vi "filter pipe.vi"(0 "omega  in":dbl[](array[numeric]), 2 "z in":cdb[](array[numeric]), 3 "upper":dbl=0.07, 5 "lower":dbl=0.01, 7 "Plot: complex plane - filter":refnum<vi>, 8 "filter using":T1(ring), 9 "interpolated omega (kHz)":dbl, 10 "filter window (kHz)":dbl=40.0 caption="(kHz)", 11 "interpolated gamma (kHz)":dbl) -> (14 "omega out":dbl[](array[numeric]), 16 "z out":cdb[](array[numeric]), 17 "center":cdb, 18 "norm":dbl, 19 "filter w (kHz)":dbl)   [LabVIEW 2010]
uses:
  <vilib>/Analysis/6fits.llb/Curve Fitting Criteria.ctl
  <vilib>/Analysis/3filter.llb/Filter Passband Type.ctl
  tale of three indices -- selector -- control.ctl
  tale of three indices -- int -- control.ctl
  linear interpolation - complex.vi
  Q -- check range -- i -- integer.vi
  command stack.vi
  generate linear region.vi
  <vilib>/Analysis/NI_AALPro.lvlib
  <vilib>/Analysis/NI_AALBase.lvlib
  <vilib>/Analysis/3filter.llb/FIR Windowed Filter (DBL).vi
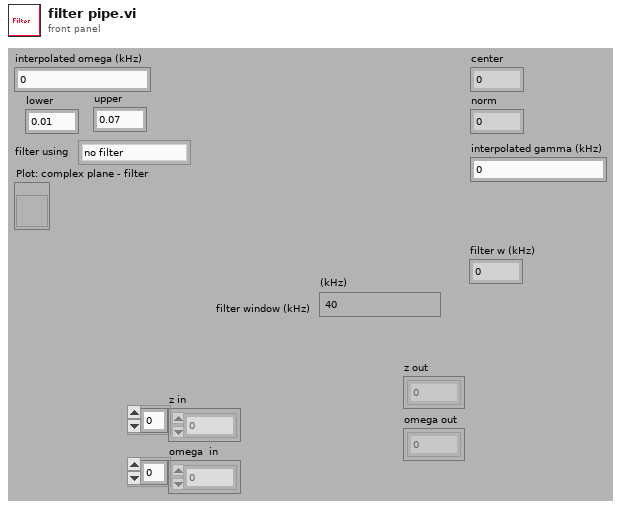
[diagram p1: front panel]
types:
  T1 = enum16{"no filter", "median", "liner fit on median", "interpolation", "smart interpolation"}
  T2 = typedef "NI_AALBase.lvlib/Filter Passband Type.ctl" = enum32{"Lowpass", "Highpass", "Bandpass", "Bandstop"}
  T3 = typedef "tale of three indices -- selector -- control.ctl" = enum16{"window right", "window left", "balance", "shrink", "broaden", "do nothing", "reset", "center right", "center left", "all left", "all right", "check"}
  T4 = typedef "NI_AALPro.lvlib/Curve Fitting Criteria.ctl" = u16
  T5 = typedef "tale of three indices -- int -- control.ctl" = cluster{"left":i32, "center":i32, "right":i32, "right most":i32, "left most":i32, "window":i32}
  T6 = typedef "comparison control.ctl" = enum16{"not a number", "above", "in range", "below"}
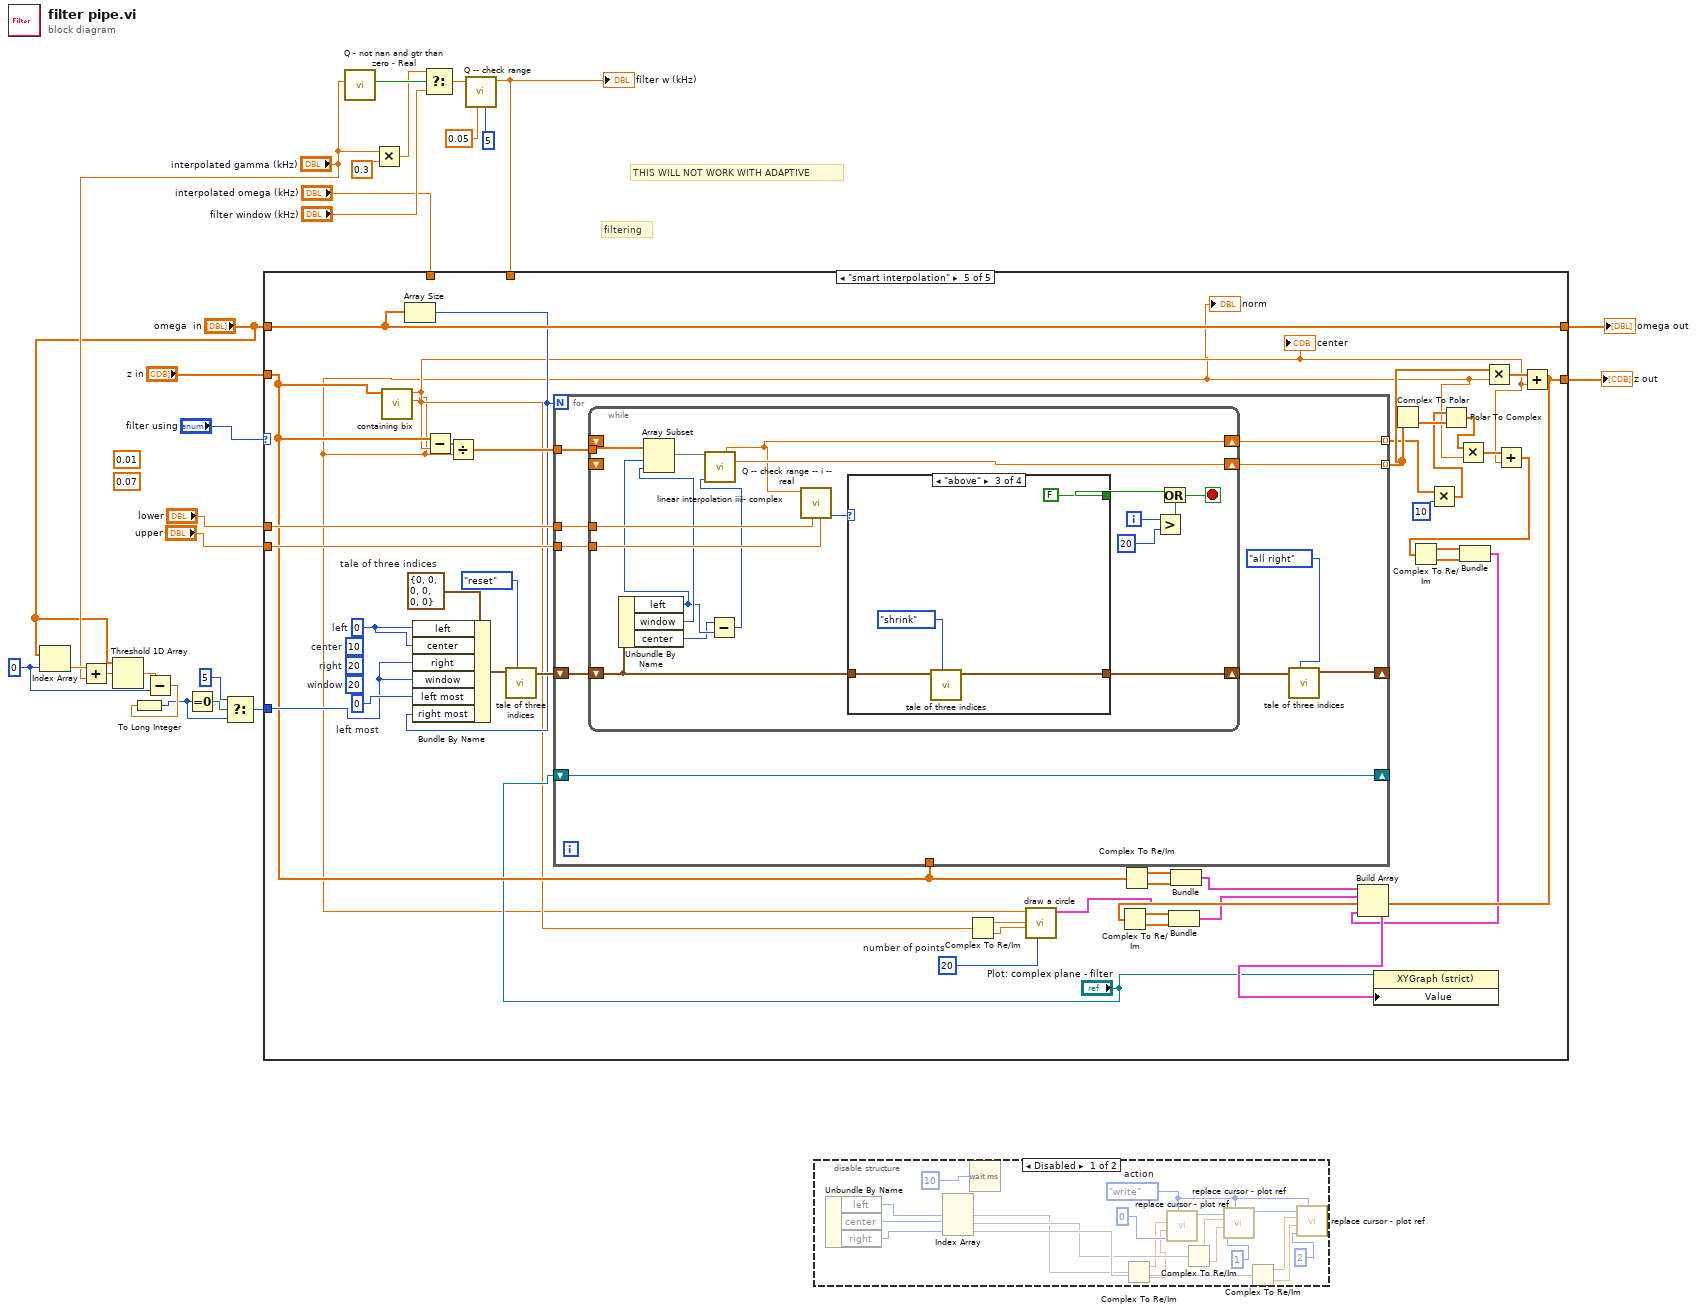
[diagram p0: block diagram]
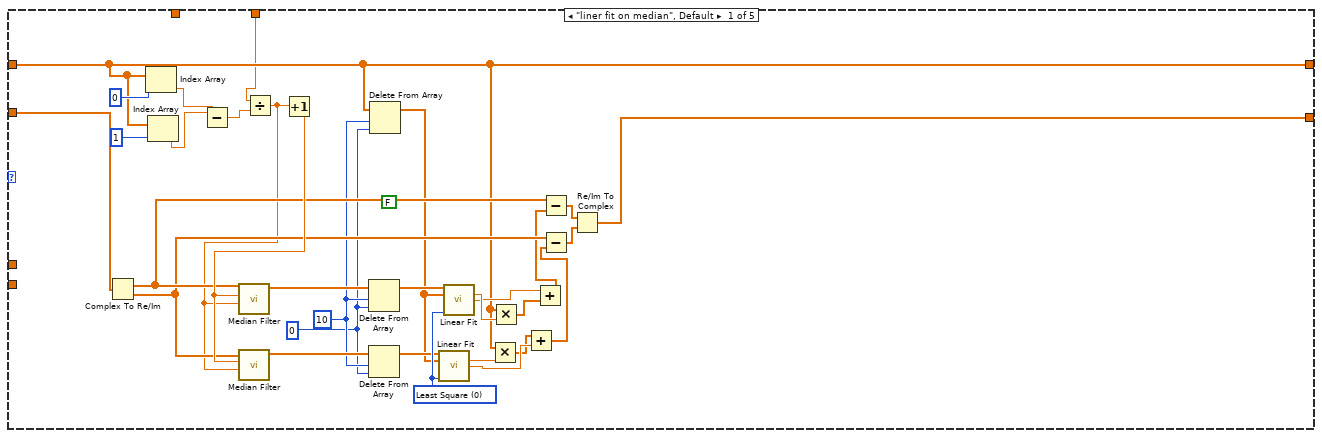
[diagram p3: hidden frame]
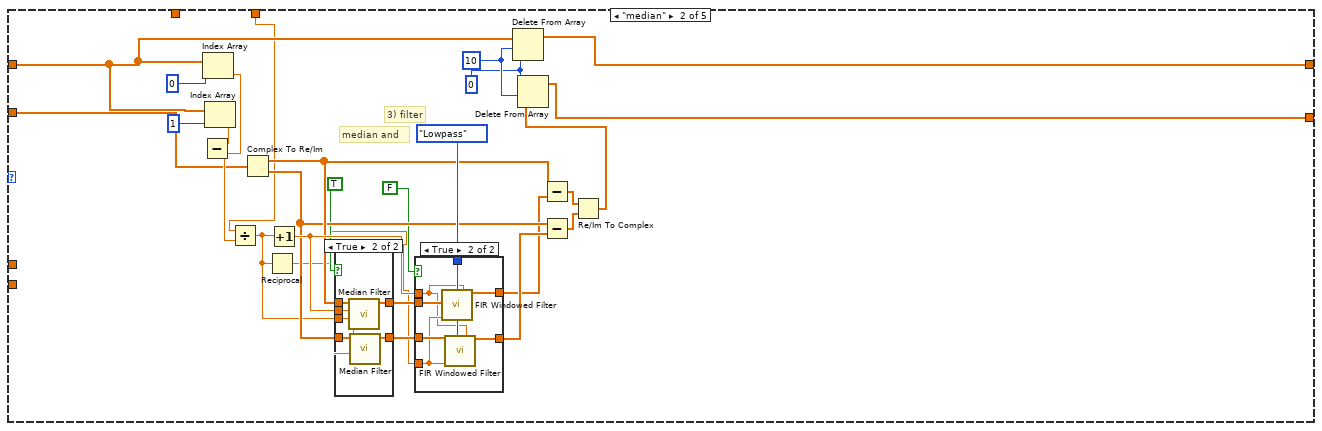
[diagram p4: hidden frame]
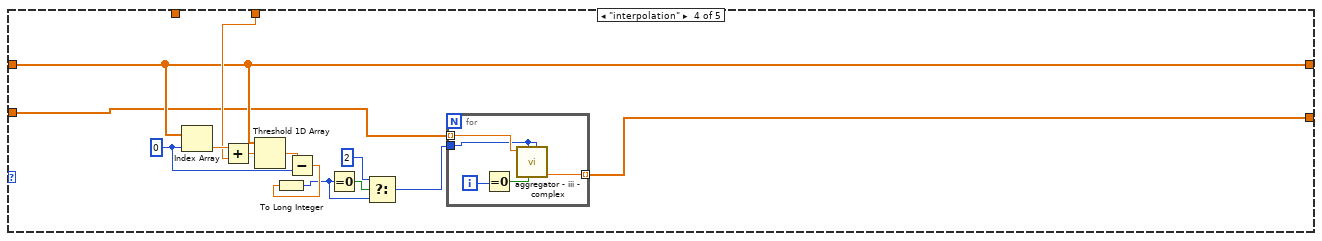
[diagram p8: hidden frame]
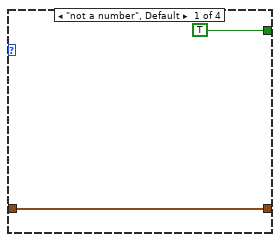
[diagram p9: hidden frame]
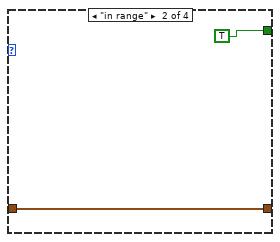
[diagram p10: hidden frame]
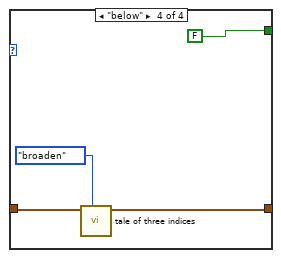
[diagram p11: hidden frame]
diagram:
  (unwired) 0.07
  (unwired) 0.01
  w10 = 0 ("index")
  # "THIS WILL NOT WORK WITH ADAPTIVE"
  # "filtering"
  n1 = Index Array(array="omega  in", index=w10) -> (element=w13:dbl)
  n2 = Add(x=w13, y="interpolated gamma (kHz)") -> (x+y=w12:dbl)
  n3 = Threshold 1D Array(2:w12, 3:"omega  in") -> (0:w11:dbl)  [unwired: 1 in]
  n4 = Subtract(x=w11, y=w10) -> (x-y=w9:dbl)
  n5 = To Long Integer(number=w9) -> (32bit integer=w6:i32)
  n6 = Equal To 0?(x=w6) -> (x = 0?=w8:bool)
  n7 = Select(t=5, s=w8, f=w6) -> (s? t:f=w4:i32)
  n8 = call "Q - not nan and gtr than zero - Real.vi"("Numeric"="interpolated gamma (kHz)") -> ("Boolean"=w22:bool)  [unwired: 9 in, 1 out]
  n9 = Multiply(x="interpolated gamma (kHz)", y=0.3) -> (x*y=w21:dbl)
  n10 = Select(t=w21, s=w22, f="filter window (kHz)") -> (s? t:f=w18:dbl)
  n11 = call "Q -- check range.vi"("upper"=5, "lower"=0.05, "number"=w18) -> ("number in range"=w17:dbl)  [unwired: 4 in, 4 out]
  "filter w (kHz)" <- w17
  n12 = case shown="\"smart interpolation\"" "filter using" {
    tunnel: "omega  in" -> [w29 w64 w103 w114 w162]
    tunnel: [w45 w65 w102 w108 w145] -> w24
    tunnel: "z in" -> [w47 w70 w102 w109 w137]
    tunnel: [w29 w61 w103 w114 w162] -> w25
    tunnel: w17 -> [w27 w58 _ w115 _]
    tunnel: "interpolated omega (kHz)" -> [_ _ _ _ _]
    tunnel: w4 -> [_ _ _ _ w153]
    tunnel: "lower" -> [_ _ _ _ w158]
    tunnel: "upper" -> [_ _ _ _ w157]
    frame "liner fit on median", Default {
      w39 = 0 ("index")
      w40 = 10 ("length")
      w46 = T4 0 items=["Least Square", "Least Absolute Residual", "Bisquare"] ("method")
      (unwired) FALSE
      n13 = Complex To Re/Im(x + iy=w47) -> (x=w50:dbl[], y=w49:dbl[])
      n14 = Index Array(array=w29, index=0) -> (element=w28:dbl)
      n15 = Index Array(array=w29, index=1) -> (element=w53:dbl)
      n16 = Subtract(x=w53, y=w28) -> (x-y=w52:dbl)
      n17 = Divide(x=w27, y=w52) -> (x/y=w48:dbl)
      n18 = Increment(x=w48) -> (x+1=w51:dbl)
      n19 = call <vilib>:"Median Filter.vi"("right rank"=w48, "left rank"=w51, "X"=w50) -> ("Filtered X"=w44:dbl[])  [unwired: 7 in, 1 out]
      n20 = call <vilib>:"Median Filter.vi"("right rank"=w48, "left rank"=w51, "X"=w49) -> ("Filtered X"=w41:dbl[])  [unwired: 7 in, 1 out]
      n21 = Delete From Array(array=w44, length=w40, index=w39) -> (array with subset deleted=w43:dbl[])  [unwired: 1 out]
      n22 = Delete From Array(array=w41, length=w40, index=w39) -> (array with subset deleted=w42:dbl[])  [unwired: 1 out]
      n23 = Delete From Array(array=w29, length=w40, index=w39) -> (array with subset deleted=w38:dbl[])  [unwired: 1 out]
      n24 = call <vilib>:"Linear Fit.vi"("Y"=w42, "X"=w38, "method"=w46) -> ("slope"=w35:dbl, "intercept"=w34:dbl)  [unwired: 8 in, 3 out]
      n25 = call <vilib>:"Linear Fit.vi"("Y"=w43, "X"=w38, "method"=w46) -> ("slope"=w36:dbl, "intercept"=w33:dbl)  [unwired: 8 in, 3 out]
      n26 = Multiply(x=w29, y=w35) -> (x*y=w32:dbl[])
      n27 = Multiply(x=w29, y=w36) -> (x*y=w37:dbl[])
      n28 = Add(x=w32, y=w34) -> (x+y=w31:dbl[])
      n29 = Add(x=w33, y=w37) -> (x+y=w30:dbl[])
      n30 = Subtract(x=w50, y=w30) -> (x-y=w57:dbl[])
      n31 = Subtract(x=w49, y=w31) -> (x-y=w56:dbl[])
      n32 = Re/Im To Complex(1:w56, 2:w57) -> (0:w45:cdb[])
    }
    frame "median" {
      w62 = 0 ("index")
      w63 = 10 ("length")
      # "median and"
      # "3) filter"
      n33 = Index Array(array=w64, index=0) -> (element=w79:dbl)
      n34 = Index Array(array=w64, index=1) -> (element=w80:dbl)
      n35 = Subtract(x=w80, y=w79) -> (x-y=w78:dbl)
      n36 = Divide(x=w58, y=w78) -> (x/y=w69:dbl)
      n37 = Complex To Re/Im(x + iy=w70) -> (x=w72:dbl[], y=w71:dbl[])
      n38 = Reciprocal(x=w69) -> (1/x=w59:dbl)
      n39 = Increment(x=w69) -> (x+1=w73:dbl)
      n40 = case shown="True" TRUE {
        tunnel: [w86 w92] -> w77
        tunnel: [w85 w91] -> w76
        tunnel: w73 -> [_ w90]
        tunnel: w72 -> [w86 w89]
        tunnel: w71 -> [w85 w88]
        tunnel: w69 -> [_ w87]
        frame False {
        }
        frame True {
          n41 = call <vilib>:"Median Filter.vi"("right rank"=w87, "left rank"=w90, "X"=w89) -> ("Filtered X"=w92:dbl[])  [unwired: 7 in, 1 out]
          n42 = call <vilib>:"Median Filter.vi"("right rank"=w87, "left rank"=w90, "X"=w88) -> ("Filtered X"=w91:dbl[])  [unwired: 7 in, 1 out]
        }
      }
      n43 = case shown="True" FALSE {
        tunnel: w77 -> [w94 w101]
        tunnel: [w94 w100] -> w60
        tunnel: w76 -> [w93 w99]
        tunnel: [w93 w98] -> w75
        tunnel: Filter_Passband_Type."Lowpass" ("filter type") -> [_ w97]
        tunnel: w59 -> [_ w96]
        tunnel: w73 -> [_ w95]
        frame False {
        }
        frame True {
          n44 = call-poly <vilib>:"FIR Windowed Filter.vi"("X"=w101, "filter type"=w97, "window parameter"=w95, "high cutoff freq: fh"=w96) -> ("Filtered X"=w100:dbl[])  [unwired: 10 in, 1 out]
          n45 = call-poly <vilib>:"FIR Windowed Filter.vi"("X"=w99, "filter type"=w97, "window parameter"=w95, "high cutoff freq: fh"=w96) -> ("Filtered X"=w98:dbl[])  [unwired: 10 in, 1 out]
        }
      }
      n46 = Delete From Array(array=w64, length=w63, index=w62) -> (array with subset deleted=w61:dbl[])  [unwired: 1 out]
      n47 = Subtract(x=w72, y=w60) -> (x-y=w84:dbl[])
      n48 = Subtract(x=w71, y=w75) -> (x-y=w83:dbl[])
      n49 = Re/Im To Complex(1:w83, 2:w84) -> (0:w66:cdb[])
      n50 = Delete From Array(array=w66, length=w63, index=w62) -> (array with subset deleted=w65:cdb[])  [unwired: 1 out]
    }
    frame "no filter" {
    }
    frame "interpolation" {
      w111 = 0 ("index")
      n51 = Index Array(array=w114, index=w111) -> (element=w116:dbl)
      n52 = Add(x=w116, y=w115) -> (x+y=w113:dbl)
      n53 = Threshold 1D Array(2:w113, 3:w114) -> (0:w112:dbl)  [unwired: 1 in]
      n54 = Subtract(x=w112, y=w111) -> (x-y=w110:dbl)
      n55 = To Long Integer(number=w110) -> (32bit integer=w105:i32)
      n56 = Equal To 0?(x=w105) -> (x = 0?=w107:bool)
      n57 = Select(t=2, s=w107, f=w105) -> (s? t:f=w104:i32)
      n58 = for {
        tunnel: w104 -> [w120]
        tunnel: w109 -> [w121] mode=indexing
        tunnel: [w117] -> w108 mode=indexing
        i -> [w119]
        n59 = Equal To 0?(x=w119) -> (x = 0?=w118:bool)
        n60 = call "aggregator - iii - complex.vi"("requested averaging interval"=w120, "first time"=w118, "requested size"=w120, "number"=w121) -> ("interpolated average"=w117:cdb)  [unwired: 3 in, 4 out]
      }
    }
    frame "smart interpolation" {
      w140 = 20  # number of points
      w156 = T5 {"left"=0, "center"=0, "right"=0, "right most"=0, "left most"=0, "window"=0}  # tale of three indices
      w155 = 0  # left most
      (unwired) 20  # window
      (unwired) 20  # right
      w154 = 0  # left
      (unwired) 10  # center
      n61 = call "containing bix.vi"("z in"=w137) -> ("norm"=w122:dbl, "center"=w130:cdb)  [unwired: 9 in]
      "center" <- w130
      "norm" <- w122
      n62 = Array Size(array=w162) -> (size(s)=w150:i32)
      n63 = Bundle By Name(cluster=w156, "left"=w154, "center"=w154, "right"=w153, "window"=w153, "left most"=w155, "right most"=w150) -> (w152:T5)
      n64 = Subtract(x=w137, y=w130) -> (x-y=w161:cdb[])
      n65 = Divide(x=w161, y=w122) -> (x/y=w160:cdb[])
      n66 = call "tale of three indices.vi"("selector"=tale_of_three_indices_--_selector_--_control."reset", "tale of three indices -- int -- control"=w152) -> ("tale of three indices -- int -- control out"=w159:T5)  [unwired: 6 in, 3 out]
      n67 = for {
        N: w150 -> [_]
        shift-right: [w167] -> _
        shift-left: w159 -> [w166]
        tunnel: [w172] -> w134 mode=indexing
        tunnel: w160 -> [w165]
        tunnel: w158 -> [w171]
        tunnel: w157 -> [w170]
        tunnel: w137 -> [_]
        shift-right: [w164] -> _
        shift-left: "Plot: complex plane - filter" -> [w164]
        tunnel: [w163] -> w125 mode=indexing
        n68 = while {
          tunnel: w165 -> [w189]
          shift-right: [w186] -> w168
          shift-left: w166 -> [w178]
          tunnel: w171 -> [w180]
          tunnel: w170 -> [w179]
          shift-right: [w173] -> w163
          shift-left: _ -> [_]
          shift-right: [w188] -> w172
          shift-left: _ -> [_]
          i -> [w183]
          stop <- w185 stop-if-true
          n69 = Unbundle By Name(w178) -> ("left"=w176:i32, "window"=w177:i32, "center"=w175:i32)
          n70 = Array Subset(array=w189, index=w176, length=w177) -> (w190:cdb[])
          n71 = Subtract(x=w175, y=w176) -> (x-y=w174:i32)
          n72 = call "linear interpolation iiii- complex.vi"("Array"=w190, "center"=w174) -> ("directed sigma"=w173:dbl, "center"=w188:cdb)  [unwired: 5 in, 7 out]
          n73 = call "Q -- check range -- i -- real.vi"("upper"=w179, "lower"=w180, "number"=w173) -> ("selector"=w187:T6)  [unwired: 6 in, 2 out]
          n74 = case shown="\"above\"" w187 {
            tunnel: [TRUE TRUE FALSE FALSE] -> w184
            tunnel: [w191 w194 w196 w199] -> w186
            tunnel: w178 -> [w191 w194 w197 w200]
            frame "not a number", Default {
            }
            frame "in range" {
            }
            frame "above" {
              n75 = call "tale of three indices.vi"("selector"=tale_of_three_indices_--_selector_--_control."shrink", "tale of three indices -- int -- control"=w197) -> ("tale of three indices -- int -- control out"=w196:T5)  [unwired: 6 in, 3 out]
            }
            frame "below" {
              n76 = call "tale of three indices.vi"("selector"=tale_of_three_indices_--_selector_--_control."broaden", "tale of three indices -- int -- control"=w200) -> ("tale of three indices -- int -- control out"=w199:T5)  [unwired: 6 in, 3 out]
            }
          }
          n77 = Greater?(x=w183, y=20) -> (0:w181:bool)
          n78 = Or(x=w184, y=w181) -> (x .or. y?=w185:bool)
        }
        n79 = call "tale of three indices.vi"("selector"=tale_of_three_indices_--_selector_--_control."all right", "tale of three indices -- int -- control"=w168) -> ("tale of three indices -- int -- control out"=w167:T5)  [unwired: 6 in, 3 out]
      }
      n80 = Complex To Re/Im(x + iy=w130) -> (x=w142:dbl, y=w141:dbl)
      n81 = call "draw a circle.vi"("number of points"=w140, "center Y"=w141, "center x"=w142, "radius"=w122) -> ("output cluster"=w139:cluster{dbl[], dbl[]})  [unwired: 7 in]
      n82 = Complex To Re/Im(x + iy=w137) -> (x=w149:dbl[], y=w148:dbl[])
      n83 = Bundle(w149, w148) -> (w144:cluster{dbl[], dbl[]})  [unwired: 1 in]
      n84 = Complex To Polar(r * e^(i*theta)=w134) -> (theta=w133:dbl[])  [unwired: 1 out]
      n85 = Multiply(x=w125, y=10) -> (x*y=w123:dbl[])
      n86 = Polar To Complex(1:w133, 2:w123) -> (0:w131:cdb[])
      n87 = Multiply(x=w131, y=w122) -> (x*y=w132:cdb[])
      n88 = Multiply(x=w134, y=w122) -> (x*y=w135:cdb[])
      n89 = Add(x=w132, y=w130) -> (x+y=w127:cdb[])
      n90 = Complex To Re/Im(x + iy=w127) -> (x=w128:dbl[], y=w129:dbl[])
      n91 = Bundle(w128, w129) -> (w126:cluster{dbl[], dbl[]})  [unwired: 1 in]
      n92 = Add(x=w135, y=w130) -> (x+y=w145:cdb[])
      n93 = Complex To Re/Im(x + iy=w145) -> (x=w147:dbl[], y=w146:dbl[])
      n94 = Bundle(w147, w146) -> (w143:cluster{dbl[], dbl[]})  [unwired: 1 in]
      n95 = Build Array(w144, w143, w139, w126) -> (w138:cluster{dbl[], dbl[]}[])
      n96 = property class="XYGraph (strict)"(reference="Plot: complex plane - filter", "Value"=w138) -> ()  [unwired: 1 in, 2 out]
    }
  }
  "z out" <- w24
  "omega out" <- w25
  n97 = disable-structure shown="Disabled" {
    frame Disabled {
      w212 = enum16{"", "read", "write"}."write"  # action
      n98 = Unbundle By Name() -> ("left"=w204:i32, "center"=w205:i32, "right"=w206:i32)  [unwired: 1 in]
      n99 = Index Array(index #1=w204, index #2=w205, index #3=w206) -> (array=w222:cdb[], element #1=w207, element #2=w217, element #3=w218)
      n100 = Wait (ms)(milliseconds to wait=10) -> ()  [unwired: 1 out]
      n101 = Complex To Re/Im(x + iy=w207) -> (x=w208:dbl, y=w209:dbl)
      n102 = call "replace cursor - plot ref.vi"("action"=w212, "cursor index"=0, "new  Y"=w209, "new X"=w208) -> ("Plot ref out"=w210:refnum<vi>)  [unwired: 5 in, 2 out]
      n103 = Complex To Re/Im(x + iy=w217) -> (x=w215:dbl, y=w216:dbl)
      n104 = call "replace cursor - plot ref.vi"("action"=w212, "cursor index"=1, "new  Y"=w216, "new X"=w215, "Plot ref in"=w210) -> ("Plot ref out"=w211:refnum<vi>)  [unwired: 4 in, 2 out]
      n105 = Complex To Re/Im(x + iy=w218) -> (x=w213:dbl, y=w214:dbl)
      n106 = call "replace cursor - plot ref.vi"("action"=w212, "cursor index"=2, "new  Y"=w214, "new X"=w213, "Plot ref in"=w211) -> ("Plot ref out"=w223:refnum<vi>)  [unwired: 4 in, 2 out]
    }
    frame Enabled {
    }
  }
